vi "targets.vi"() -> (0 "objects":refnum<vi>[](array[refnum]), 2 "shperes":refnum<vi>[](array[refnum]), 3 "Scene:New Object":refnum<vi>)   [LabVIEW 2011]
uses:
  <vilib>/picture/3D Picture Control/NI_3D Picture Control.lvlib
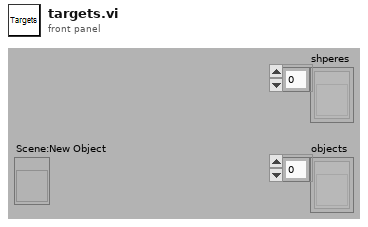
[diagram p1: front panel]
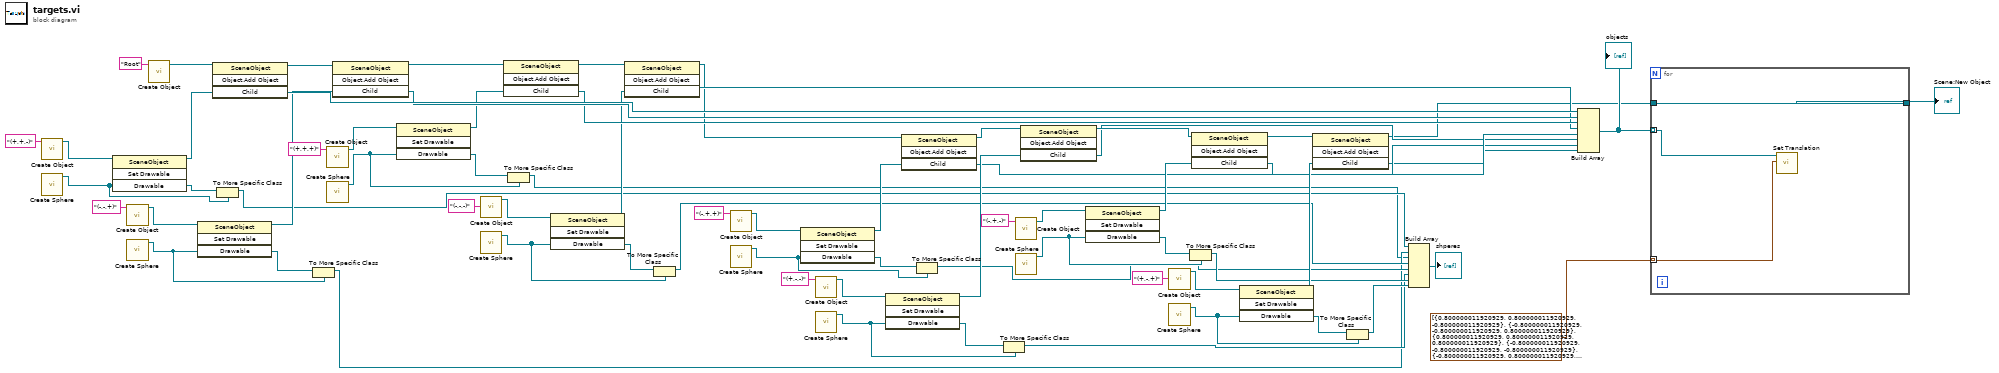
[diagram p0: block diagram]
diagram:
  n1 = call <vilib>:"Create Object.vi"("Name"="(+,+,-)") -> ("Scene:New Object"=w68:refnum<vi>)  [unwired: 9 in, 1 out]
  n2 = call <vilib>:"Create Sphere.vi"() -> ("New Sphere Refnum"=w24:refnum<vi>)  [unwired: 10 in, 1 out]
  n3 = invoke class="SceneObject" method="Set Drawable"(reference=w68, "Drawable"=w24) -> (reference out=w56:refnum<vi>, "Drawable"=w25:refnum<vi>)  [unwired: 2 in, 2 out]
  n4 = call <vilib>:"Create Object.vi"("Name"="(-,-,+)") -> ("Scene:New Object"=w66:refnum<vi>)  [unwired: 9 in, 1 out]
  n5 = call <vilib>:"Create Sphere.vi"() -> ("New Sphere Refnum"=w22:refnum<vi>)  [unwired: 10 in, 1 out]
  n6 = call <vilib>:"Create Object.vi"("Name"="Root") -> ("Scene:New Object"=w69:refnum<vi>)  [unwired: 9 in, 1 out]
  n7 = invoke class="SceneObject" method="Set Drawable"(reference=w66, "Drawable"=w22) -> (reference out=w55:refnum<vi>, "Drawable"=w23:refnum<vi>)  [unwired: 2 in, 2 out]
  n8 = invoke class="SceneObject" method="Object.Add Object"(reference=w69, "Child"=w56) -> (reference out=w67:refnum<vi>, "Child"=w61:refnum<vi>)  [unwired: 2 in, 2 out]
  n9 = To More Specific Class(target class=w24, reference=w25) -> (specific class reference=w4:refnum<vi>)  [unwired: 1 in, 1 out]
  n10 = To More Specific Class(target class=w22, reference=w23) -> (specific class reference=w3:refnum<vi>)  [unwired: 1 in, 1 out]
  n11 = call <vilib>:"Create Object.vi"("Name"="(+,+,+)") -> ("Scene:New Object"=w64:refnum<vi>)  [unwired: 9 in, 1 out]
  n12 = call <vilib>:"Create Sphere.vi"() -> ("New Sphere Refnum"=w20:refnum<vi>)  [unwired: 10 in, 1 out]
  n13 = invoke class="SceneObject" method="Object.Add Object"(reference=w67, "Child"=w55) -> (reference out=w65:refnum<vi>, "Child"=w60:refnum<vi>)  [unwired: 2 in, 2 out]
  n14 = invoke class="SceneObject" method="Set Drawable"(reference=w64, "Drawable"=w20) -> (reference out=w54:refnum<vi>, "Drawable"=w21:refnum<vi>)  [unwired: 2 in, 2 out]
  n15 = call <vilib>:"Create Object.vi"("Name"="(-,-,-)") -> ("Scene:New Object"=w63:refnum<vi>)  [unwired: 9 in, 1 out]
  n16 = call <vilib>:"Create Sphere.vi"() -> ("New Sphere Refnum"=w18:refnum<vi>)  [unwired: 10 in, 1 out]
  n17 = invoke class="SceneObject" method="Object.Add Object"(reference=w65, "Child"=w54) -> (reference out=w62:refnum<vi>, "Child"=w59:refnum<vi>)  [unwired: 2 in, 2 out]
  n18 = To More Specific Class(target class=w20, reference=w21) -> (specific class reference=w2:refnum<vi>)  [unwired: 1 in, 1 out]
  n19 = invoke class="SceneObject" method="Set Drawable"(reference=w63, "Drawable"=w18) -> (reference out=w53:refnum<vi>, "Drawable"=w19:refnum<vi>)  [unwired: 2 in, 2 out]
  n20 = invoke class="SceneObject" method="Object.Add Object"(reference=w62, "Child"=w53) -> (reference out=w45:refnum<vi>, "Child"=w58:refnum<vi>)  [unwired: 2 in, 2 out]
  n21 = To More Specific Class(target class=w18, reference=w19) -> (specific class reference=w5:refnum<vi>)  [unwired: 1 in, 1 out]
  n22 = call <vilib>:"Create Object.vi"("Name"="(-,+,+)") -> ("Scene:New Object"=w51:refnum<vi>)  [unwired: 9 in, 1 out]
  n23 = call <vilib>:"Create Sphere.vi"() -> ("New Sphere Refnum"=w16:refnum<vi>)  [unwired: 10 in, 1 out]
  n24 = invoke class="SceneObject" method="Set Drawable"(reference=w51, "Drawable"=w16) -> (reference out=w47:refnum<vi>, "Drawable"=w17:refnum<vi>)  [unwired: 2 in, 2 out]
  n25 = call <vilib>:"Create Object.vi"("Name"="(+,-,-)") -> ("Scene:New Object"=w50:refnum<vi>)  [unwired: 9 in, 1 out]
  n26 = call <vilib>:"Create Sphere.vi"() -> ("New Sphere Refnum"=w14:refnum<vi>)  [unwired: 10 in, 1 out]
  n27 = invoke class="SceneObject" method="Set Drawable"(reference=w50, "Drawable"=w14) -> (reference out=w40:refnum<vi>, "Drawable"=w15:refnum<vi>)  [unwired: 2 in, 2 out]
  n28 = invoke class="SceneObject" method="Object.Add Object"(reference=w45, "Child"=w47) -> (reference out=w44:refnum<vi>, "Child"=w39:refnum<vi>)  [unwired: 2 in, 2 out]
  n29 = To More Specific Class(target class=w16, reference=w17) -> (specific class reference=w6:refnum<vi>)  [unwired: 1 in, 1 out]
  n30 = To More Specific Class(target class=w14, reference=w15) -> (specific class reference=w7:refnum<vi>)  [unwired: 1 in, 1 out]
  n31 = call <vilib>:"Create Object.vi"("Name"="(-,+,-)") -> ("Scene:New Object"=w49:refnum<vi>)  [unwired: 9 in, 1 out]
  n32 = call <vilib>:"Create Sphere.vi"() -> ("New Sphere Refnum"=w12:refnum<vi>)  [unwired: 10 in, 1 out]
  n33 = invoke class="SceneObject" method="Object.Add Object"(reference=w44, "Child"=w40) -> (reference out=w43:refnum<vi>, "Child"=w38:refnum<vi>)  [unwired: 2 in, 2 out]
  n34 = invoke class="SceneObject" method="Set Drawable"(reference=w49, "Drawable"=w12) -> (reference out=w46:refnum<vi>, "Drawable"=w13:refnum<vi>)  [unwired: 2 in, 2 out]
  n35 = call <vilib>:"Create Object.vi"("Name"="(+,-,+)") -> ("Scene:New Object"=w48:refnum<vi>)  [unwired: 9 in, 1 out]
  n36 = call <vilib>:"Create Sphere.vi"() -> ("New Sphere Refnum"=w10:refnum<vi>)  [unwired: 10 in, 1 out]
  n37 = To More Specific Class(target class=w12, reference=w13) -> (specific class reference=w8:refnum<vi>)  [unwired: 1 in, 1 out]
  n38 = invoke class="SceneObject" method="Object.Add Object"(reference=w43, "Child"=w46) -> (reference out=w42:refnum<vi>, "Child"=w37:refnum<vi>)  [unwired: 2 in, 2 out]
  n39 = invoke class="SceneObject" method="Set Drawable"(reference=w48, "Drawable"=w10) -> (reference out=w41:refnum<vi>, "Drawable"=w11:refnum<vi>)  [unwired: 2 in, 2 out]
  n40 = invoke class="SceneObject" method="Object.Add Object"(reference=w42, "Child"=w41) -> (reference out=w35:refnum<vi>, "Child"=w36:refnum<vi>)  [unwired: 2 in, 2 out]
  n41 = To More Specific Class(target class=w10, reference=w11) -> (specific class reference=w9:refnum<vi>)  [unwired: 1 in, 1 out]
  n42 = Build Array(w4, w3, w2, w5, w6, w7, w8, w9) -> (→"shperes":refnum<vi>[])
  n43 = Build Array(w61, w60, w59, w58, w39, w38, w37, w36) -> (w57:refnum<vi>[])
  "objects" <- w57
  n44 = for {
    tunnel: w57 -> [w71] mode=indexing
    tunnel: cluster{"X":sgl, "Y":sgl, "Z":sgl}[] [{"X"=0.8, "Y"=0.8, "Z"=-0.8}, {"X"=-0.8, "Y"=-0.8, "Z"=0.8}, {"X"=0.8, "Y"=0.8, "Z"=0.8}, {"X"=-0.8, "Y"=-0.8, "Z"=-0.8}, {"X"=-0.8, "Y"=0.8, "Z"=0.8}, {"X"=0.8, "Y"=-0.8, "Z"=-0.8}, {"X"=-0.8, "Y"=0.8, "Z"=-0.8}, {"X"=0.8, "Y"=-0.8, "Z"=0.8}] -> [w73] mode=indexing
    tunnel: w35 -> [w72]
    tunnel: [w72] -> w34
    n45 = call <vilib>:"Set Translation.vi"("Translation"=w73, "Scene Object"=w71) -> ()  [unwired: 8 in, 2 out]
  }
  "Scene:New Object" <- w34
